vi "Adjust Escala.vi"(8 "error in (no error)":errorcluster, 10 "Escala":dbl) -> (0 "error out":errorcluster, 2 "Escala String":string)   [LabVIEW 2015]
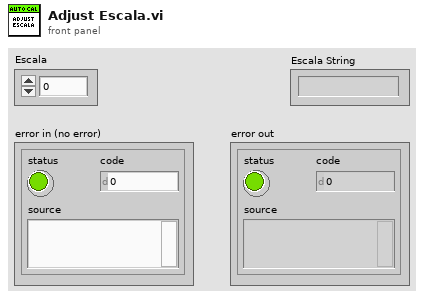
[diagram p1: front panel]
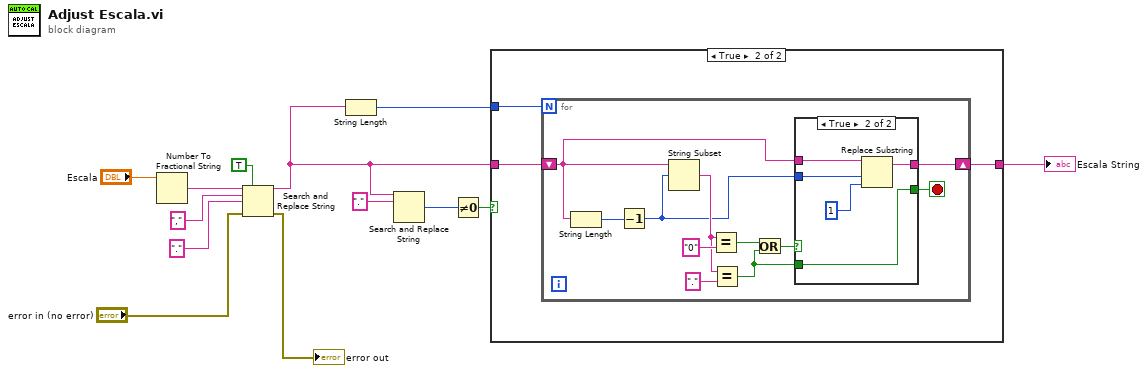
[diagram p0: block diagram]
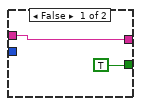
[diagram p3: hidden frame]
diagram:
  n1 = Number To Fractional String(number="Escala") -> (F-format string=w13:string)  [unwired: 3 in]
  n2 = Search and Replace String(replace all?=TRUE ("replace all? (F)"), input string=w13, search string=",", replace string="." ("replace string (\"\")"), error in="error in (no error)") -> (result string=w4:string, error out=→"error out":errorcluster)  [unwired: 3 in, 2 out]
  n3 = String Length(string=w4) -> (length=w8:i32)
  n4 = Search and Replace String(input string=w4, search string=".") -> (number of replacements=w2:i32)  [unwired: 6 in, 3 out]
  n5 = Not Equal To 0?(x=w2) -> (x != 0?=w1:bool)
  n6 = case shown="True" w1 {
    tunnel: w8 -> [_ w17]
    tunnel: [w14 w16] -> w7
    tunnel: w4 -> [w14 w15]
    frame False {
    }
    frame True {
      n7 = for {
        N: w17 -> [_]
        shift-right: [w22] -> w16
        shift-left: w15 -> [w19]
        stop <- w21 stop-if-true
        n8 = String Length(string=w19) -> (length=w20:i32)
        n9 = Decrement(x=w20) -> (x-1=w23:i32)
        n10 = String Subset(string=w19, offset (0)=w23) -> (substring=w27:string)  [unwired: 1 in]
        n11 = Equal?(x=w27, y="0") -> (x = y?=w24:bool)
        n12 = Equal?(x=w27, y=".") -> (x = y?=w18:bool)
        n13 = Or(x=w24, y=w18) -> (x .or. y?=w25:bool)
        n14 = case shown="True" w25 {
          tunnel: w19 -> [w30 w35]
          tunnel: w23 -> [_ w34]
          tunnel: [w30 w33] -> w22
          tunnel: [TRUE w31] -> w21
          tunnel: w18 -> [_ w31]
          frame False {
          }
          frame True {
            n15 = Replace Substring(2:1 ("length (len. of substring)"), 3:w34, 5:w35) -> (1:w33:string)  [unwired: 1 in, 1 out]
          }
        }
      }
    }
  }
  "Escala String" <- w7
